vi "setWaveform_AS.vi"(1 "error in (no error)":errorcluster, 2 "Frequency (1000 Hz)":dbl=1000000.0, 3 "Enum":enum16{"Triangle", "Sine"}(ring), 4 "VISA resource name":refnum<visa-resource-name>="GPIB0::4::INSTR") -> (0 "error out":errorcluster)   [LabVIEW 2016]
doc: "Shows how to configure then create an arbitrary waveform."
uses:
  Instance           2 56Saved   Agilent 33XXX Series Generate Arbitrary Waveform .vi
  Instance           1 56Saved   Agilent 33XXX Series Generate Arbitrary Waveform .vi
  Agilent 33XXX Series.lvlib
panel:
  in  "Gain (1.0)":dbl=5.0
  in  "Offset (0 V)":dbl
  # "(c) 2005 - 2013 National Instruments.  ALL RIGHTS RESERVED."
  # "To edit the Arbitrary Waveform, use the Simulate Arbitrary Signal on the block diagram; or choose from the options below."
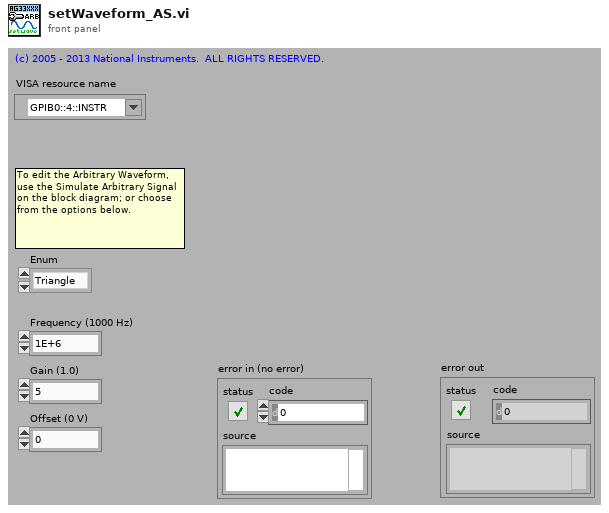
[diagram p1: front panel]
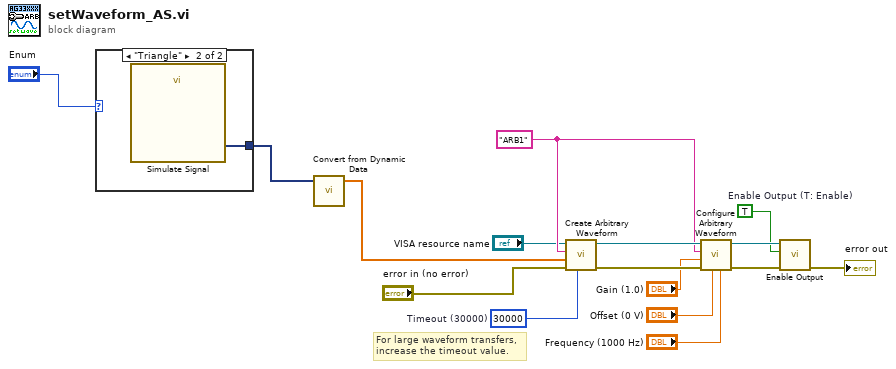
[diagram p0: block diagram]
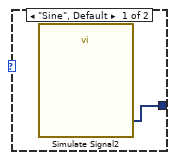
[diagram p2: hidden frame]
diagram:
  w11 = "ARB1" ("Arbitrary Waveform Name")
  w8 = u32 30000  # Timeout (30000)
  w12 = TRUE  # Enable Output (T: Enable)
  # "For large waveform transfers, increase the timeout value."
  n1 = case shown="\"Triangle\"" "Enum" {
    tunnel: [w17 w18] -> w6
    frame "Sine", Default {
      n2 = call "Simulate Signal2"() -> ("Sine"=w17:dynamicdata)  [unwired: 14 in, 1 out]
    }
    frame "Triangle" {
      n3 = call "Simulate Signal"() -> ("Triangle"=w18:dynamicdata)  [unwired: 14 in, 1 out]
    }
  }
  n4 = call "Convert from Dynamic Data"("Dynamic Data Type"=w6) -> ("Array"=w7:dbl[])  [unwired: 3 in]
  n5 = call "Create Arbitrary Waveform.vi"("Timeout (10000)"=w8, "error in (no error)"="error in (no error)", "Arbitrary Waveform Data"=w7, "Arbitrary Waveform Name (\"ARB1\")"=w11, "VISA resource name"="VISA resource name") -> ("error out"=w15:errorcluster, "VISA resource name out"=w16:refnum<visa-resource-name>)  [unwired: 5 in]
  n6 = call "Configure Arbitrary Waveform.vi"("Frequency (1000 Hz)"="Frequency (1000 Hz)", "Offset (0.00 V)"="Offset (0 V)", "error in (no error)"=w15, "Gain (1.0)"="Gain (1.0)", "Arbitrary Waveform Name (\"ARB1\")"=w11, "VISA resource name"=w16) -> ("error out"=w13:errorcluster, "VISA resource name out"=w14:refnum<visa-resource-name>)  [unwired: 4 in]
  n7 = call "Enable Output.vi"("error in (no error)"=w13, "Enable Output  (T: Enable)"=w12, "VISA resource name"=w14) -> ("error out"=→"error out":errorcluster)  [unwired: 7 in, 1 out]
